vi "Run Step.vi"(8 "error in (no error)":errorcluster, 9 "result allocation":T1, 10 "parameters":T1, 11 "Conditional Jump Step in":refnum<class "Conditional Jump Step.lvclass">) -> (0 "error out":errorcluster, 1 "results":T1, 2 "parameter allocation":T1, 3 "Conditional Jump Step out":refnum<class "Conditional Jump Step.lvclass">)   [LabVIEW 2015, in "Conditional Jump Step.lvclass"]
uses:
  Conditional Jump Step.lvclass
  <vilib>/NI/Tag Bus/table/data table.ctl
  Conditional Jump Step.lvclass/Conditional Jump Step.ctl
  <vilib>/NI/Tag Bus/table/data polymorphs/read one/read Boolean.vi
  <vilib>/NI/Tag Bus/table/data table.lvlib
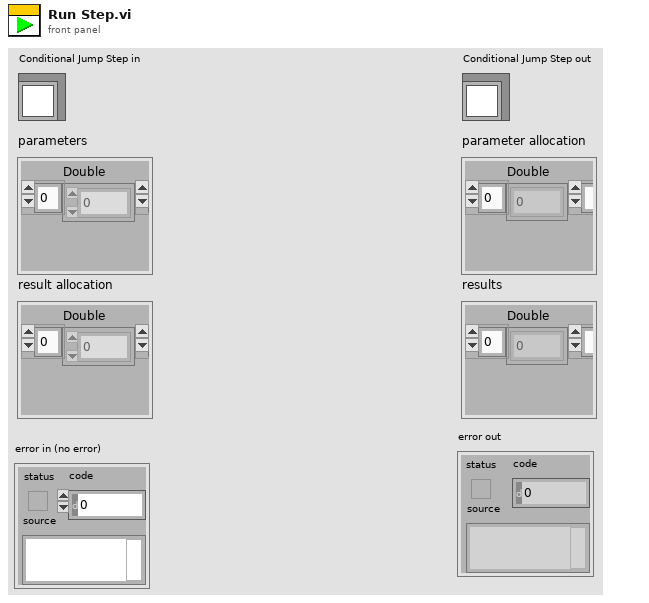
[diagram p1: front panel]
types:
  T1 = typedef "tag bus.lvlib/data table.lvlib/data table.ctl" = cluster{"Double":dbl[], "Single":sgl[], "I64":i64[], "I32":i32[], "I16":i16[], "I8":i8[], "U64":u64[], "U32":u32[], "U16":u16[], "U8":u8[], "Boolean":bool[], "String":string[], "Array of Double":cluster{"DBL Array":dbl[]}[], "Array of Single":cluster{"SGL Array":sgl[]}[], "Array of I64":cluster{"I64 Array":i64[]}[], "Array of I32":cluster{"I32 Array":i32[]}[], "Array of I16":cluster{"I16 Array":i16[]}[], "Array of I8":cluster{"I8 Array":i8[]}[], "Array of U64":cluster{"U64 Array":u64[]}[], "Array of U32":cluster{"U32 Array":u32[]}[], "Array of U16":cluster{"U16 Array":u16[]}[], "Array of U8":cluster{"U8 Array":u8[]}[], "Array of Boolean":cluster{"Boolean Array":bool[]}[], "Array of String":cluster{"String Array":string[]}[]}
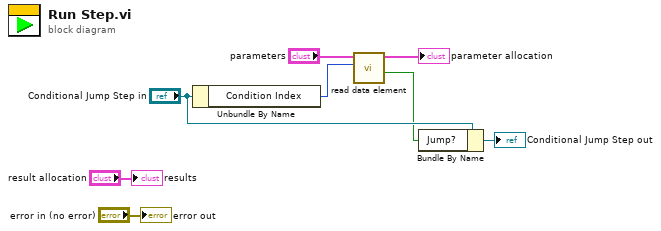
[diagram p0: block diagram]
diagram:
  n1 = Unbundle By Name("Conditional Jump Step in") -> ("Condition Index"=w2:i32)
  n2 = call-poly <vilib>:"read data element.vi"("index"=w2, "data table in"="parameters") -> ("value"=w3:bool, "data table out"=→"parameter allocation":T1)  [unwired: 8 in]
  n3 = Bundle By Name(cluster="Conditional Jump Step in", "Jump?"=w3) -> (→"Conditional Jump Step out":refnum<class "Conditional Jump Step.lvclass">)
  "error out" <- "error in (no error)"
  "results" <- "result allocation"
